vi "test lvjson get.vi"(8 "error in (no error)":errorcluster) -> (0 "error out":errorcluster)   [LabVIEW 2019, in "labview_json_tests.lvlib"]
uses:
  lib/Element Type.ctl
  labview_json_tests.lvlib
  lib/labview_json.lvlib
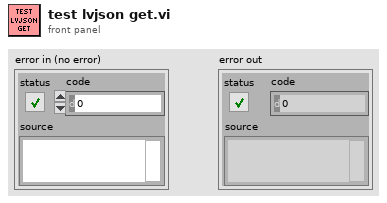
[diagram p1: front panel]
types:
  T1 = typedef "labview_json.lvlib/Element Type.ctl" = enum8{"NULL", "OBJECT", "ARRAY", "BOOL", "INT", "UINT", "FLOAT", "STRING"}
  T2 = typedef "labview_json.lvlib/Element.ctl" = cluster{"Key":string, "Type":T1, "Value":variant}
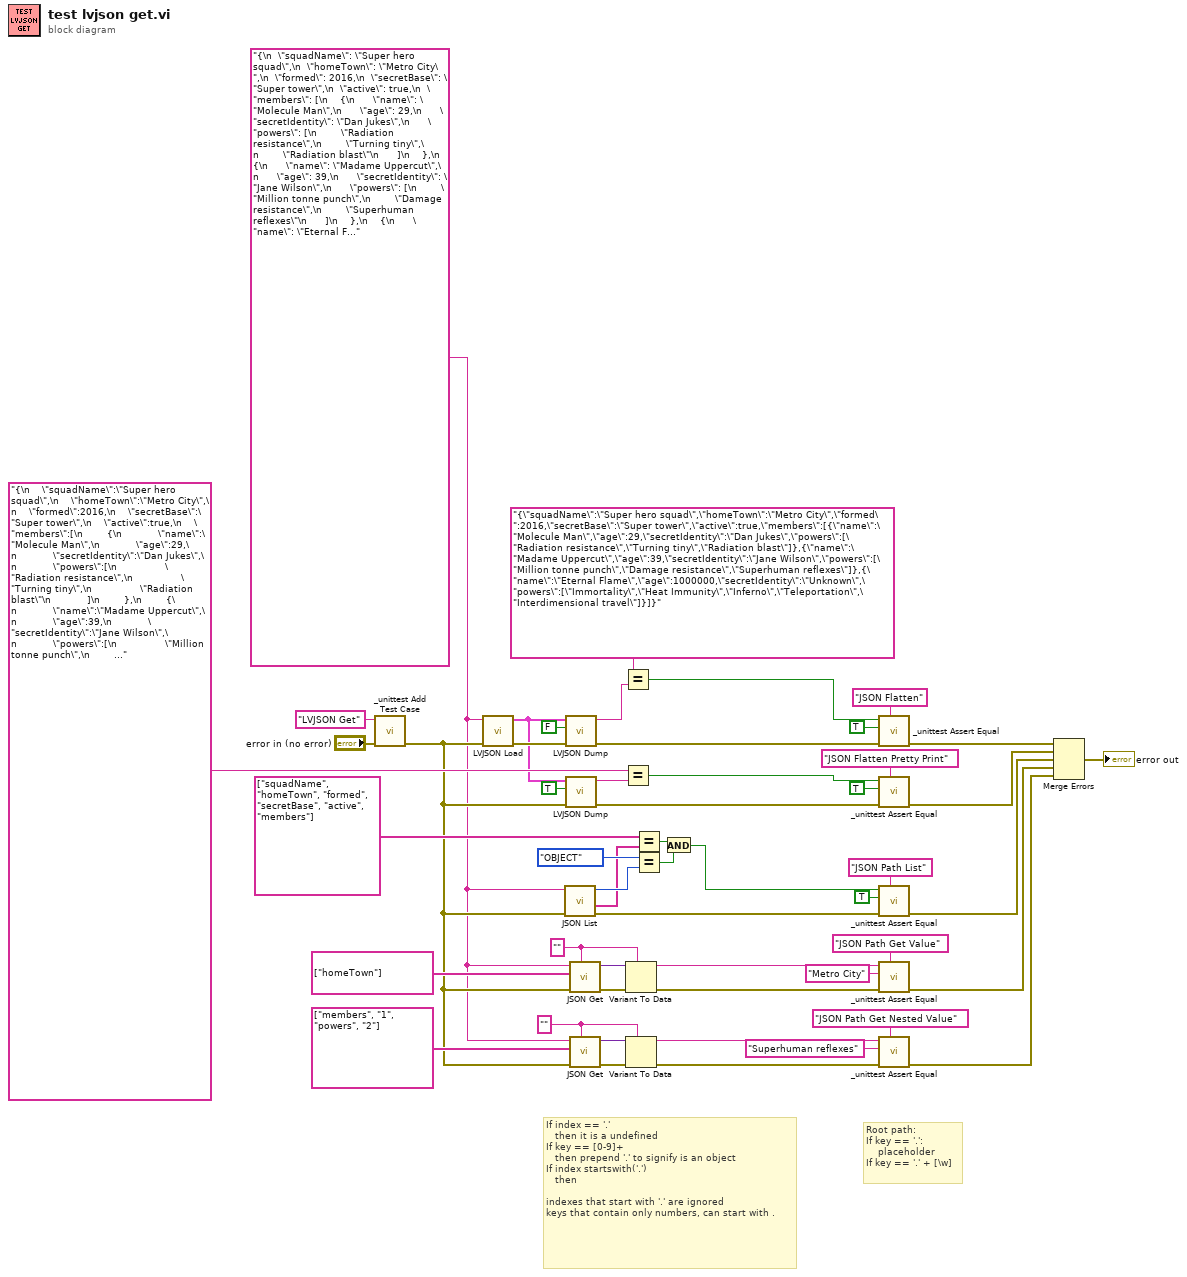
[diagram p0: block diagram]
diagram:
  w8 = ""
  w6 = ""
  w1 = "{\n  \"squadName\": \"Super hero squad\",\n  \"homeTown\": \"Metro City\",\n  \"formed\": 2016,\n  \"secretBase\": \"Super tower\",\n  \"active\": true,\n  \"members\": [\n    {\n      \"name\": \"Molecule Man\",\n      \"age\": 29,\n      \"secretIdentity\": \"Dan Jukes\",\n      \"powers\": [\n        \"Radiation resistance\",\n        \"Turning tiny\",\n        \"Radiation blast\"\n      ]\n    },\n    {\n      \"name\": \"Madame Uppercut\",\n      \"age\": 39,\n      \"secretIdentity\": \"Jane Wilson\",\n      \"powers\": [\n        \"Million tonne punch\",\n        \"Damage resistance\",\n        \"Superhuman reflexes\"\n      ]\n    },\n    {\n      \"name\": \"Eternal Flame\",\n      \"age\": 1000000,\n      \"secretIdentity\": \"Unknown\",\n      \"powers\": [\n        \"Immortality\",\n        \"Heat Immunity\",\n        \"Inferno\",\n        \"Teleportation\",\n        \"Interdimensional travel\"\n      ]\n    }\n  ]\n}"
  # "Root path:\nIf key == '.':\n    placeholder\nIf key == '.' + [\\w]"
  # "If index == '.'\n   then it is a undefined\nIf key == [0-9]+\n   then prepend '.' to signify is an object\nIf index startswith('.')\n   then\n\nindexes that start with '.' are ignored\nkeys that contain only numbers, can start with ."
  n1 = call "_unittest Add Test Case.vi"("error in (no error)"="error in (no error)", "Test Case"="LVJSON Get") -> ("error out"=w5:errorcluster)  [unwired: 9 in]
  n2 = call "LVJSON Load.vi"("error in (no error)"=w5, "JSON in"=w1) -> ("error out"=w46:errorcluster, "Root Element out"=w17:T2)  [unwired: 8 in]
  n3 = call "JSON List.vi"("error in (no error)"=w5, "JSON in"=w1) -> ("error out"=w4:errorcluster, "Keys/Indexes"=w2:string[], "Type"=w3:T1)  [unwired: 6 in, 1 out]
  n4 = call "LVJSON Dump.vi"("error in (no error)"=w46, "Pretty Print? (F)"=FALSE, "Root Element in"=w17) -> ("error out"=w45:errorcluster, "JSON out"=w43:string)  [unwired: 6 in, 1 out]
  n5 = call "LVJSON Dump.vi"("error in (no error)"=w5, "Pretty Print? (F)"=TRUE, "Root Element in"=w17) -> ("error out"=w35:errorcluster, "JSON out"=w37:string)  [unwired: 6 in, 1 out]
  n6 = call "JSON Get.vi"("Default"=w8, "error in (no error)"=w5, "Root Path ([]=Root)"=string[] ["homeTown"] ("JSON Path"), "JSON in"=w1) -> ("error out"=w13:errorcluster, "Value"=w9:variant)  [unwired: 5 in, 1 out]
  n7 = call "JSON Get.vi"("Default"=w6, "error in (no error)"=w5, "Root Path ([]=Root)"=string[] ["members", "1", "powers", "2"] ("JSON Path"), "JSON in"=w1) -> ("error out"=w15:errorcluster, "Value"=w7:variant)  [unwired: 5 in, 1 out]
  n8 = Equal?(x="{\"squadName\":\"Super hero squad\",\"homeTown\":\"Metro City\",\"formed\":2016,\"secretBase\":\"Super tower\",\"active\":true,\"members\":[{\"name\":\"Molecule Man\",\"age\":29,\"secretIdentity\":\"Dan Jukes\",\"powers\":[\"Radiation resistance\",\"Turning tiny\",\"Radiation blast\"]},{\"name\":\"Madame Uppercut\",\"age\":39,\"secretIdentity\":\"Jane Wilson\",\"powers\":[\"Million tonne punch\",\"Damage resistance\",\"Superhuman reflexes\"]},{\"name\":\"Eternal Flame\",\"age\":1000000,\"secretIdentity\":\"Unknown\",\"powers\":[\"Immortality\",\"Heat Immunity\",\"Inferno\",\"Teleportation\",\"Interdimensional travel\"]}]}" ("JSON"), y=w43) -> (x = y?=w41:bool)
  n9 = Equal?(x="{\n    \"squadName\":\"Super hero squad\",\n    \"homeTown\":\"Metro City\",\n    \"formed\":2016,\n    \"secretBase\":\"Super tower\",\n    \"active\":true,\n    \"members\":[\n        {\n            \"name\":\"Molecule Man\",\n            \"age\":29,\n            \"secretIdentity\":\"Dan Jukes\",\n            \"powers\":[\n                \"Radiation resistance\",\n                \"Turning tiny\",\n                \"Radiation blast\"\n            ]\n        },\n        {\n            \"name\":\"Madame Uppercut\",\n            \"age\":39,\n            \"secretIdentity\":\"Jane Wilson\",\n            \"powers\":[\n                \"Million tonne punch\",\n                \"Damage resistance\",\n                \"Superhuman reflexes\"\n            ]\n        },\n        {\n            \"name\":\"Eternal Flame\",\n            \"age\":1000000,\n            \"secretIdentity\":\"Unknown\",\n            \"powers\":[\n                \"Immortality\",\n                \"Heat Immunity\",\n                \"Inferno\",\n                \"Teleportation\",\n                \"Interdimensional travel\"\n            ]\n        }\n    ]\n}" ("JSON"), y=w37) -> (x = y?=w39:bool)
  n10 = Variant To Data(error in=w13, type=w8, Variant=w9) -> (data=w10:string, error out=w11:errorcluster)
  n11 = Variant To Data(error in=w15, type=w6, Variant=w7) -> (data=w20:string, error out=w19:errorcluster)
  n12 = Equal?(x=string[] ["squadName", "homeTown", "formed", "secretBase", "active", "members"], y=w2) -> (x = y?=w28:bool)
  n13 = Equal?(x=Element_Type."OBJECT", y=w3) -> (x = y?=w27:bool)
  n14 = And(x=w28, y=w27) -> (x .and. y?=w26:bool)
  n15 = call "_unittest Assert Equal.vi"("Message"="JSON Flatten", "error in (no error)"=w45, "Expected Value"=TRUE, "Actual Value"=w41) -> ("error out"=w50:errorcluster)  [unwired: 7 in]
  n16 = call "_unittest Assert Equal.vi"("Message"="JSON Flatten Pretty Print", "error in (no error)"=w35, "Expected Value"=TRUE, "Actual Value"=w39) -> ("error out"=w33:errorcluster)  [unwired: 7 in]
  n17 = call "_unittest Assert Equal.vi"("Message"="JSON Path List", "error in (no error)"=w4, "Expected Value"=TRUE, "Actual Value"=w26) -> ("error out"=w32:errorcluster)  [unwired: 7 in]
  n18 = call "_unittest Assert Equal.vi"("Message"="JSON Path Get Value", "error in (no error)"=w11, "Expected Value"="Metro City", "Actual Value"=w10) -> ("error out"=w23:errorcluster)  [unwired: 7 in]
  n19 = call "_unittest Assert Equal.vi"("Message"="JSON Path Get Nested Value", "error in (no error)"=w19, "Expected Value"="Superhuman reflexes", "Actual Value"=w20) -> ("error out"=w16:errorcluster)  [unwired: 7 in]
  n20 = Merge Errors(w50, w33, w32, w23, w16) -> (→"error out":errorcluster)
